vi "Load DAC Configuration.vi"(8 "error in":errorcluster, 10 "Config File refnum in":T1, 11 "DAC HTS dU in":refnum<class "DAC HTS dU.lvclass">) -> (0 "error out":errorcluster, 2 "Config File refnum out":T1, 3 "DAC HTS dU out":refnum<class "DAC HTS dU.lvclass">)   [LabVIEW 2019, in "DAC.lvlib" / "DAC HTS dU.lvclass"]
uses:
  DAC HTS dU.lvclass
  <vilib>/Utility/config.llb/Config Data RefNum.ctl
  DAC.lvclass
  <vilib>/Utility/config.llb/NI_LVConfig.lvlib
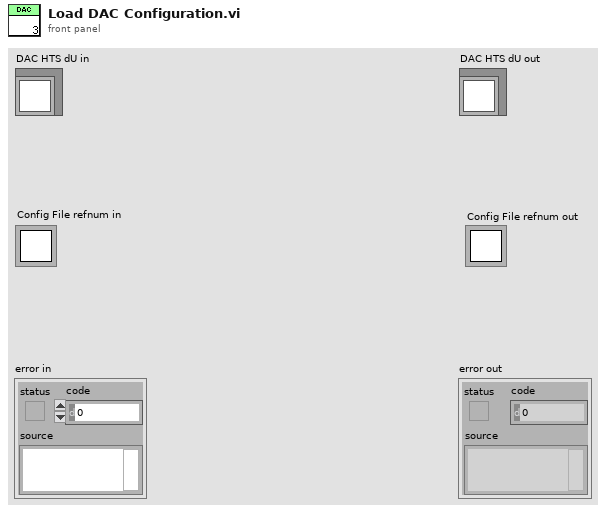
[diagram p1: front panel]
types:
  T1 = typedef "NI_LVConfig.lvlib/Config Data RefNum.ctl" = refnum<k1>
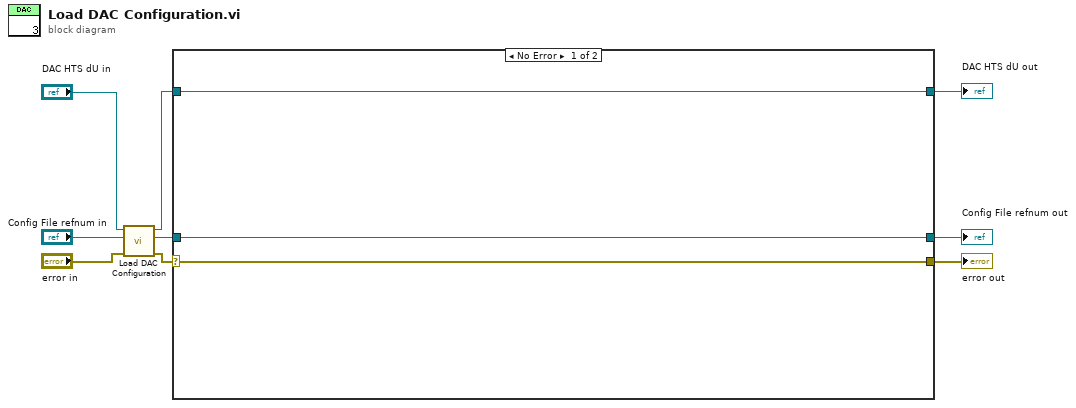
[diagram p0: block diagram]
diagram:
  n1 = call-parent "Load DAC Configuration.vi"("error in"="error in", "Config File refnum in"="Config File refnum in", "DAC in"="DAC HTS dU in") -> ("error out"=w4:errorcluster, "Config File refnum out"=w5:T1, "DAC out"=w6:refnum<class "DAC HTS dU.lvclass">)  [unwired: 6 in]
  n2 = case shown="No Error" w4 {
    selector: w4 -> [w10 w15]
    tunnel: [w10 w15] -> w1
    tunnel: [w12 w14] -> w3
    tunnel: w6 -> [w12 w14]
    tunnel: w5 -> [w11 w13]
    tunnel: [w11 w13] -> w2
    frame No Error {
    }
    frame Error {
    }
  }
  "error out" <- w1
  "DAC HTS dU out" <- w3
  "Config File refnum out" <- w2
